vi "SSL Detection Frame Robots Kalman Estimator VelCmd.vi"(0 "Lado":enum16{"Esquerdo", "Direito"}(ring) caption="Enum", 5 "Time Stamp":timestamp, 6 "our_robots":bool=TRUE, 7 "Life Time":dbl=1.0, 10 "our_robots":T1[](array[typedef]), 11 "Robots":T6[](array[typedef]) {"height" format="%+4.3f"; "pixel_y" format="%+4.3f"; "pixel_x" format="%+4.3f"; "orientation" format="%+4.3f"; "y" format="%+4.3f"; "confidence" format="%4.3f"; "x" format="%+4.3f"}) -> (3 "Robots Out":T6[](array[typedef]) {"height" format="%+4.3f"; "pixel_y" format="%+4.3f"; "pixel_x" format="%+4.3f"; "orientation" format="%+4.3f"; "y" format="%+4.3f"; "confidence" format="%4.3f"; "x" format="%+4.3f"})   [LabVIEW 2018]
uses:
  Controls/SSL Detection Robot.ctl
  <vilib>/Analysis/Matrix/Datatypes/RealMatrix.ctl
  Controls/AI Robot.ctl
  Controls/Functions Enum.ctl
  Controls/AttackerStates.ctl
  Controls/PathDests.ctl
  Controls/PathDest.ctl
  <vilib>/Analysis/coordinate.llb/Wrap Angle (scalar).vi
  <vilib>/Analysis/_algsub.llb/Real Vector Norm.vi
  <vilib>/Analysis/Matrix/Numeric/Conversions/Array To Matrix - RA.vi
  <vilib>/Analysis/Matrix/Numeric/Subtract/Subtract - RM,RM.vi
  <vilib>/Analysis/NI_AALPro.lvlib
  <vilib>/Analysis/Matrix/NI_Matrix.lvlib
  <vilib>/Analysis/NI_AAL_Angle.lvlib
panel:
  in  "Robots Out 2":T8(array[cluster]) {"Detection Robot"."height" format="%+4.3f"; "Detection Robot"."pixel_y" format="%+4.3f"; "Detection Robot"."pixel_x" format="%+4.3f"; "Detection Robot"."orientation" format="%+4.3f"; "Detection Robot"."y" format="%+4.3f"; "Detection Robot"."confidence" format="%4.3f"; "Detection Robot"."x" format="%+4.3f"}
  out "A-B":dbl[][](array[numeric])
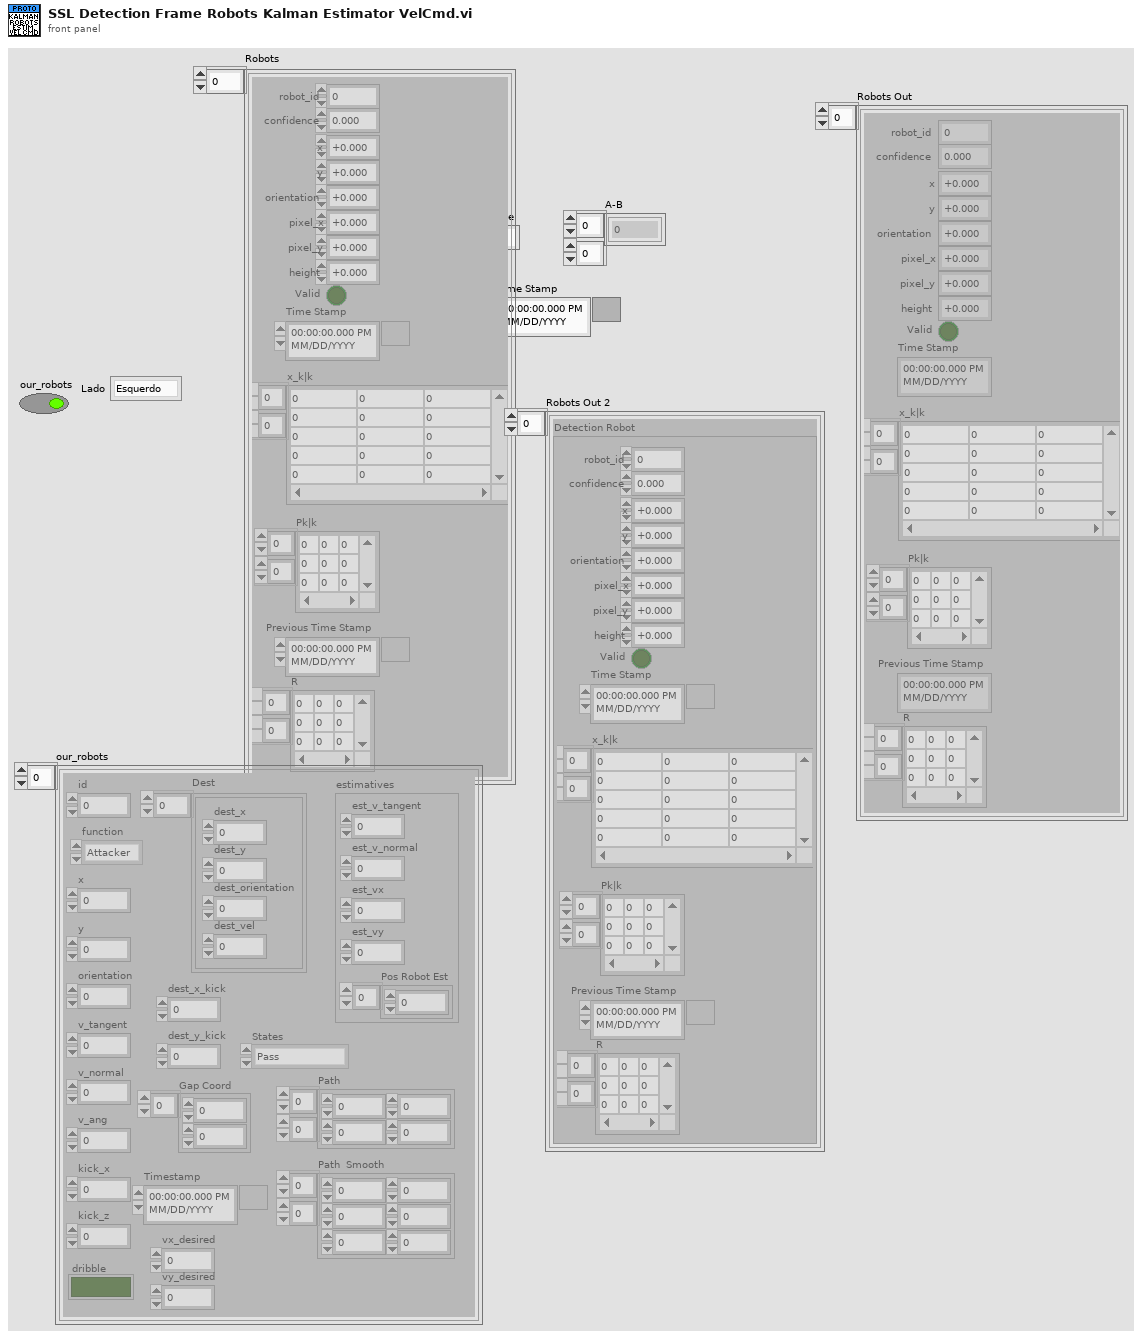
[diagram p1: front panel]
types:
  T1 = typedef "AI Robot.ctl" = cluster{"id":u32, "function":T2, "x":dbl, "y":dbl, "orientation":dbl, "v_tangent":dbl, "v_normal":dbl, "v_ang":dbl, "kick_x":dbl, "kick_z":dbl, "dribble":bool, "Timestamp":timestamp, "estimatives":cluster{"est_v_tangent":dbl, "est_v_normal":dbl, "est_vx":dbl, "est_vy":dbl, "Pos Robot Est":dbl[]}, "dest_x_kick":dbl, "dest_y_kick":dbl, "Gap Coord":dbl[], "States":T3, "Path ":dbl[][], "Path  Smooth":dbl[][], "Dest":T4, "vx_desired":dbl, "vy_desired":dbl}
  T2 = typedef "Functions Enum.ctl" = enum16{"2nd Striker", "Attacker", "Goalie", "Defender", "Striker", "Goto 0", "Dummy", "Kicker", "ZigZag 0", "ZigZag 1", "ZigZag 2", "ZigZag 3", "ZigZag 4", "ZigZag 5", "ZigZag 6", "ZigZag 7", "ZigZag 8", ""}
  T3 = typedef "AttackerStates.ctl" = enum16{"Pass", "GoToTangent", "BallGetting", "GoToKick", ""}
  T4 = typedef "PathDests.ctl" = T5[]
  T5 = typedef "PathDest.ctl" = cluster{"dest_x":dbl, "dest_y":dbl, "dest_orientation":dbl, "dest_vel":dbl}
  T6 = typedef "SSL Detection Robot.ctl" = cluster{"x":sgl, "robot_id":u32, "confidence":sgl, "y":sgl, "orientation":sgl, "pixel_x":sgl, "pixel_y":sgl, "height":sgl, "Valid":bool, "Time Stamp":timestamp, "x_k|k":T7, "Pk|k":T7, "Previous Time Stamp":timestamp, "R":T7}
  T7 = typedef "NI_Matrix.lvlib/RealMatrix.ctl" = dbl[][]
  T8 = cluster{"Detection Robot":T6, "Real Matrix (Column Vector)":T7, "Pk|k":T7}[]
  T9 = cluster{"Detection Robot":T6, "Real Matrix (Column Vector)":T7, "Pk|k":T7}
  T10 = cluster{"Detection Robot out":T6, "x_k|k":T7, "Pk|k":T7}
  T11 = typedef "SSL Detection Robot.ctl" = cluster{"x":sgl, "robot_id":u32, "confidence":sgl, "y":sgl, "orientation":sgl, "pixel_x":sgl, "pixel_y":sgl, "height":sgl, "Valid":bool, "Time Stamp":timestamp, "x_k|k":T7, "Pk|k":T7}
  T12 = cluster{"Detection Robot":T11, "Real Matrix (Column Vector)":T7, dbl[][]}
  T13 = cluster{"Detection Robot out":T6, "x_k|k":T7, "Pk|k":T7}[]
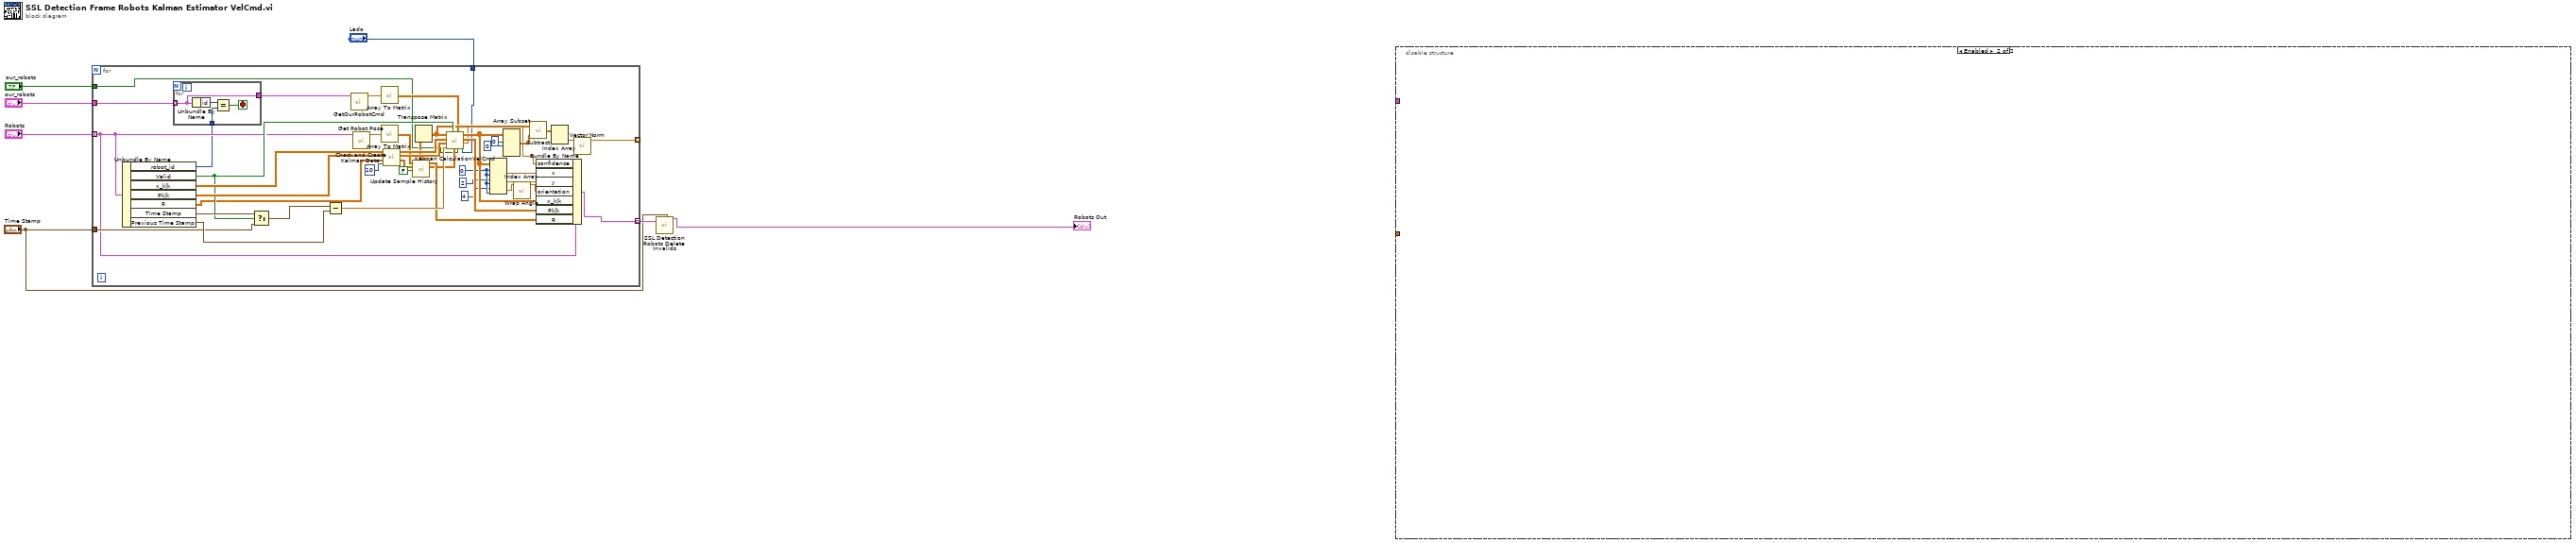
[diagram p0: block diagram]
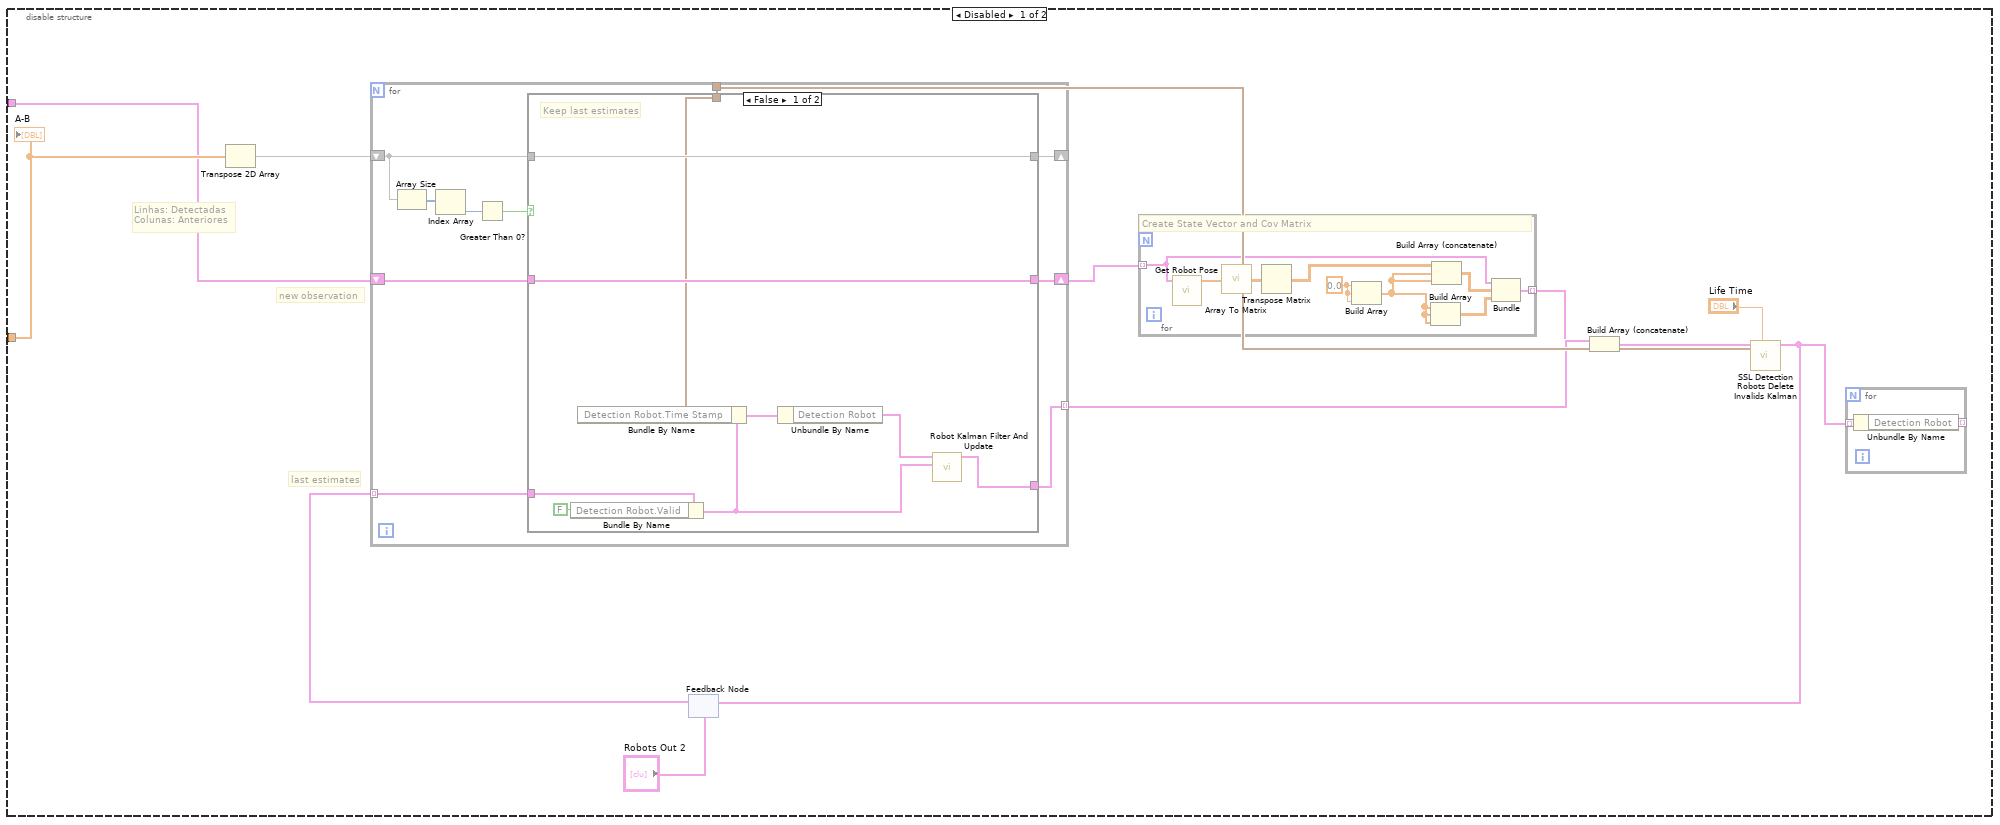
[diagram p2: hidden frame]
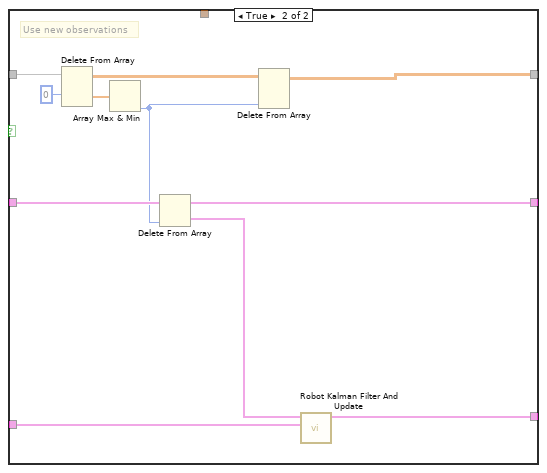
[diagram p3: hidden frame]
diagram:
  n1 = for {
    tunnel: "Robots" -> [w34] mode=indexing
    tunnel: [w52] -> _ mode=indexing
    tunnel: [w16] -> w6 mode=indexing
    tunnel: "Time Stamp" -> [w37]
    tunnel: "our_robots" -> [w15]
    tunnel: "our_robots" -> [w10]
    tunnel: "Lado" -> [w9]
    w30 = 0 ("index (row)")
    n2 = Unbundle By Name(w34) -> ("robot_id"=w14:u32, "Valid"=w35:bool, "x_k|k"=w44:T7, "Pk|k"=w42:T7, "R"=w27:T7, "Time Stamp"=w38:timestamp, "Previous Time Stamp"=w40:timestamp)
    n3 = for {
      tunnel: w15 -> [w53] mode=indexing
      tunnel: w14 -> [w54]
      tunnel: [w53] -> w13
      stop <- w56 stop-if-true
      n4 = Unbundle By Name(w53) -> ("id"=w55:u32)
      n5 = Equal?(x=w55, y=w54) -> (x = y?=w56:bool)
    }
    n6 = Select(t=w38, s=w35, f=w37) -> (s? t:f=w36:timestamp)
    n7 = Subtract(x=w36, y=w40) -> (x-y=w39:dbl)
    n8 = call "GetOurRobotCmd.vi"("Robot"=w13) -> ("Vel"=w12:dbl[])  [unwired: 10 in]
    n9 = call "Get Robot Pose.vi"("Detection Robot"=w34) -> ("Pose"=w46:sgl[])  [unwired: 10 in]
    n10 = call-poly <vilib>:"Array To Matrix.vi"("Real 1D Array"=w12) -> ("Real Matrix (Column Vector)"=w11:T7)
    n11 = call-poly <vilib>:"Array To Matrix.vi"("Real 1D Array"=w46) -> ("Real Matrix (Column Vector)"=w23:T7)
    n12 = call "Check and Create Kalman Data.vi"("Variance Memory"=10, "R"=w27, "Pk"=w42, "x_k"=w44) -> ("R out"=w26:T7, "Pk out"=w41:T7, "x_k out"=w43:T7)  [unwired: 5 in]
    n13 = call "Update Sample History.vi"("Ball?"=FALSE, "R in"=w26, "Sample"=w23) -> ("covariance matrix V"=w21:T7, "R out"=w22:T7, "Sample Unwrapped"=w20:T7)  [unwired: 6 in]
    n14 = Transpose Matrix(1:w20) -> (0:w24:T7)
    n15 = call "Kalman CalculationVelCmd.vi"("Lado"=w9, "our_robots"=w10, "u_k"=w11, "R"=w21, "Use Observation"=w35, "intervalo"=w39, "Pk-1|k-1"=w41, "x_k-1|k-1"=w43, "z_k"=w24) -> ("Conf"=w17:dbl, "Pk|k"=w45:T7, "x_k|k"=w33:T7)
    n16 = Index Array(array=w33, index (row) #1=w30, index (col) #1=w30, index (row) #2=2 ("disabled index (col)"), index (col) #2=w30, index (row) #3=4 ("disabled index (col)"), index (col) #3=w30) -> (element #1=w32:dbl, element #2=w31:dbl, element #3=w19:dbl)
    n17 = Array Subset(array=w33, index (row)=0 ("row 1"), length (row)=0 ("row N")) -> (w51:T7)  [unwired: 2 in]
    n18 = call-poly <vilib>:"Wrap Angle.vi"("angle in"=w19) -> ("angle out"=w18:dbl)  [unwired: 9 in, 1 out]
    n19 = call-poly <vilib>:"Subtract.vi"("Real Matrix B"=w51, "Real Matrix A"=w24) -> ("A - B"=w48:T7)
    n20 = Bundle By Name(cluster=w34, "confidence"=w17, "x"=w32, "y"=w31, "orientation"=w18, "x_k|k"=w33, "Pk|k"=w45, "R"=w22) -> (w16:T6)
    n21 = Index Array(array=w48) -> (element=w47:dbl[])  [unwired: 2 in]
    n22 = call-poly <vilib>:"Vector Norm.vi"("Input Vector"=w47) -> ("norm"=w52:dbl)  [unwired: 9 in, 1 out]
  }
  n23 = call "SSL Detection Robots Delete Invalids.vi"("Now"="Time Stamp", "Robots In"=w6) -> ("Robots Out"=→"Robots Out":T6[])  [unwired: 9 in]
  n24 = disable-structure shown="Enabled" {
    disable-tunnel: _ -> [w65 _]
    disable-tunnel: _ -> [w64 _]
    frame Disabled {
      # "Linhas: Detectadas\nColunas: Anteriores"
      # "last estimates"
      # "new observation"
      n25 = Transpose 2D Array(2D array=w65) -> (transposed array=w66:dbl[][])
      n26 = feedback #1("Robots Out 2") -> (w58:T8)
      n27 = for {
        shift-right: [w88] -> _
        shift-left: w66 -> [w84]
        shift-right: [w87] -> w63
        shift-left: w64 -> [w89]
        tunnel: [w86] -> w62 mode=indexing
        tunnel: w58 -> [w85] mode=indexing
        tunnel: [w80] -> w67
        n28 = Array Size(array=w84) -> (size(s)=w82:i32[])
        n29 = Index Array(array=w82) -> (element=w81:i32)  [unwired: 1 in]
        n30 = Greater Than 0?(x=w81) -> (x > 0?=w83:bool)
        n31 = case shown="False" w83 {
          tunnel: w84 -> [w98 w109]
          tunnel: w89 -> [w97 w106]
          tunnel: [w98 w104] -> w88
          tunnel: [w97 w102] -> w87
          tunnel: [w93 w101] -> w86
          tunnel: w85 -> [w92 w99]
          tunnel: w80 -> [w95 _]
          frame False {
            # "Keep last estimates"
            n32 = Bundle By Name(cluster=w92, "Detection Robot.Valid"=FALSE ("Detection Ball.Valid")) -> (w90:T9)
            n33 = Bundle By Name(cluster=w90, "Detection Robot.Time Stamp"=w95) -> (w94:T9)
            n34 = Unbundle By Name(w94) -> ("Detection Robot"=w91:T6)
            n35 = call "Robot Kalman Filter And Update.vi"("Cluster in"=w90, "Detection Robot"=w91) -> ("Cluster out"=w93:T10)  [unwired: 9 in]
          }
          frame True {
            # "Use new observations"
            n36 = Delete From Array(array=w109, index (row)=0) -> (deleted portion=w107:dbl[], array with subset deleted=w105:dbl[][])  [unwired: 2 in]
            n37 = Array Max & Min(array=w107) -> (min index (indices)=w103:i32)  [unwired: 3 out]
            n38 = Delete From Array(array=w106, index=w103) -> (deleted portion=w100:T11, array with subset deleted=w102:T11[])  [unwired: 1 in]
            n39 = Delete From Array(array=w105, index (col)=w103) -> (array with subset deleted=w104:dbl[][])  [unwired: 2 in, 1 out]
            n40 = call "Robot Kalman Filter And Update.vi"("Cluster in"=w99, "Detection Robot"=w100) -> ("Cluster out"=w101:T10)  [unwired: 9 in]
          }
        }
      }
      n41 = for {
        tunnel: w63 -> [w72] mode=indexing
        tunnel: [w75] -> w61 mode=indexing
        w79 = 0.0 ("element")
        # "Create State Vector and Cov Matrix"
        n42 = call "Get Robot Pose.vi"("Detection Robot"=w72) -> ("Pose"=w74:sgl[])  [unwired: 10 in]
        n43 = call-poly <vilib>:"Array To Matrix.vi"("Real 1D Array"=w74) -> ("Real Matrix (Column Vector)"=w73:T7)
        n44 = Transpose Matrix(1:w73) -> (0:w71:T7)
        n45 = Build Array(w79, w79, w79) -> (w78:dbl[])
        n46 = Build Array(w78, w78, w78) -> (w77:dbl[][])
        n47 = Build Array (concatenate)(w71, w78, w78) -> (w76:T7)
        n48 = Bundle("Detection Robot"=w72, "Real Matrix (Column Vector)"=w76, w77) -> (w75:T12)  [unwired: 1 in]
      }
      n49 = Build Array (concatenate)(w62, w61) -> (w57:T13)
      n50 = call "SSL Detection Robots Delete Invalids Kalman.vi"("Now"=w67, "Life Time"="Life Time", "Robots In"=w57) -> ("Robots Out"=w60:T8)  [unwired: 8 in]
      n51 = feedback-in #1(w60) -> ()
      n52 = for {
        tunnel: w60 -> [w70] mode=indexing
        tunnel: [w69] -> _ mode=indexing
        n53 = Unbundle By Name(w70) -> ("Detection Robot"=w69:T6)
      }
      "A-B" <- w65
    }
    frame Enabled {
    }
  }
